vi "Update Calibration (Months).vi"(5 "New Calibration Password":string, 6 "Remote Timeout (300,000 ms)":u32=300000, 7 "Calibration Password":string, 8 "error in (no error)":errorcluster, 9 "Interval in Months (-1)":i32=-1, 10 "Calibration Date":timestamp, 11 "Resource in":refnum<k20>) -> (0 "error out":errorcluster, 2 "Detailed Result":string, 3 "Resource out":refnum<k20>)   [LabVIEW 2014, in "nisyscfg.lvlib"]
doc: "Updates the external calibration date in months for a device. You can only use this VI to update calibration information if the Supports Calibration Write property is TRUE."
uses:
  nisyscfg.lvlib
  C:/Program Files (x86)/National Instruments/LabVIEW 2014/resource/objmgr/nisysapi.rc
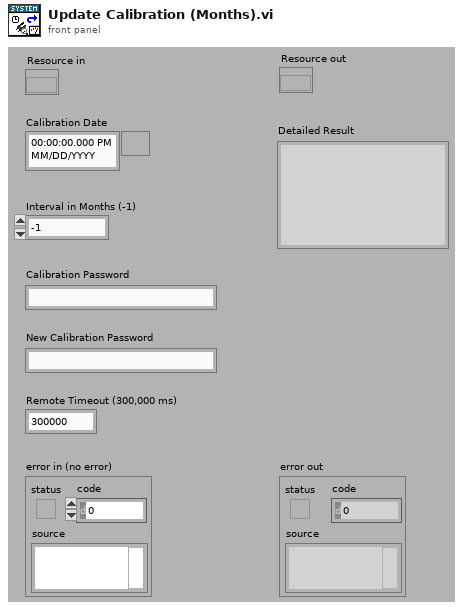
[diagram p1: front panel]
types:
  T1 = typedef "LVDateTimeRec.ctl" = cluster{"fractional second":dbl, "second":i32, "minute":i32, "hour":i32, "day of month":i32, "month":i32, "year":i32, "day of week":i32, "day of year":i32, "DST":i32}
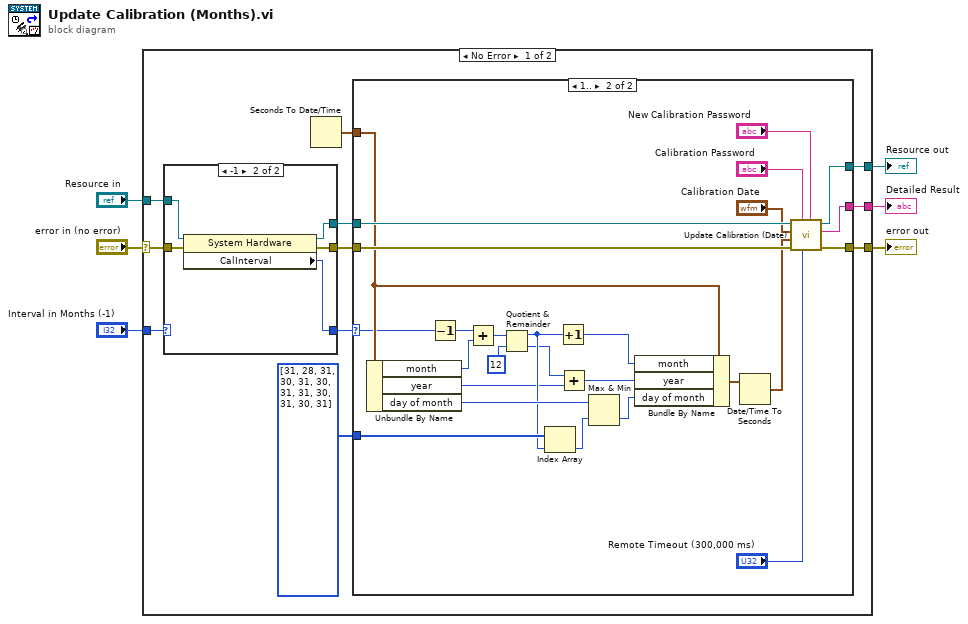
[diagram p0: block diagram]
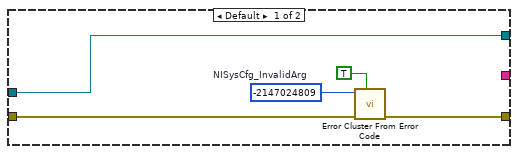
[diagram p2: hidden frame]
diagram:
  n1 = case shown="No Error" "error in (no error)" {
    selector: "error in (no error)" -> [w15 w58]
    tunnel: [w11 w58] -> w6
    tunnel: "Resource in" -> [w16 w57]
    tunnel: [w9 w57] -> w3
    tunnel: "Interval in Months (-1)" -> [w17 _]
    tunnel: [w10 _] -> w1
    frame No Error {
      n2 = case shown="-1" w17 {
        selector: w17 -> [w51 _]
        tunnel: w16 -> [w49 w56]
        tunnel: w15 -> [w50 w55]
        tunnel: [w50 w54] -> w13
        tunnel: [w51 w53] -> w14
        tunnel: [w49 w52] -> w12
        frame Default {
        }
        frame -1 {
          n3 = property class="System Hardware"(reference=w56, error in=w55) -> (reference out=w52:refnum<k20>, error out=w54:errorcluster, "CalInterval"=w53:i32)
        }
      }
      n4 = Seconds To Date/Time() -> (date time rec=w8:T1)  [unwired: 2 in]
      n5 = case shown="1.." w14 {
        selector: w14 -> [_ w31]
        tunnel: w13 -> [w20 w43]
        tunnel: w12 -> [w22 w41]
        tunnel: [w19 w36] -> w11
        tunnel: [_ w35] -> w10
        tunnel: [w22 w34] -> w9
        tunnel: w8 -> [_ w33]
        tunnel: i32[] [31, 28, 31, 30, 31, 30, 31, 31, 30, 31, 30, 31] -> [_ w32]
        frame Default {
          w18 = -2147024809  # NISysCfg_InvalidArg
          n6 = call "Error Cluster From Error Code.vi"("show call chain? (False)"=TRUE, "error in (no error)"=w20, "error code (0)"=w18) -> ("error out"=w19:errorcluster)  [unwired: 6 out]
        }
        frame 1.. {
          n7 = Unbundle By Name(w33) -> ("month"=w48:i32, "year"=w24:i32, "day of month"=w46:i32)
          n8 = Decrement(x=w31) -> (x-1=w30:i32)
          n9 = Add(x=w30, y=w48) -> (x+y=w28:i32)
          n10 = Quotient & Remainder(x=w28, y=12) -> (x-y*floor(x/y)=w27:i32, floor(x/y)=w25:i32)
          n11 = Index Array(array=w32, index=w27) -> (element=w47:i32)
          n12 = Increment(x=w27) -> (x+1=w26:i32)
          n13 = Add(x=w25, y=w24) -> (x+y=w23:i32)
          n14 = Max & Min(x=w46, y=w47) -> (min(x,y)=w45:i32)  [unwired: 1 out]
          n15 = Bundle By Name(cluster=w33, "month"=w26, "year"=w23, "day of month"=w45) -> (w44:T1)
          n16 = Date/Time To Seconds(2:w44) -> (0:w42:timestamp)  [unwired: 1 in]
          n17 = call "Update Calibration (Date).vi"("New Calibration Password"="New Calibration Password", "Remote Timeout (300,000 ms)"="Remote Timeout (300,000 ms)", "Calibration Password"="Calibration Password", "error in (no error)"=w43, "Calibration Due Date"=w42, "Calibration Date"="Calibration Date", "Resource in"=w41) -> ("error out"=w36:errorcluster, "Detailed Result"=w35:string, "Resource out"=w34:refnum<k20>)  [unwired: 2 in]
        }
      }
    }
    frame Error {
    }
  }
  "error out" <- w6
  "Resource out" <- w3
  "Detailed Result" <- w1
